vi "jeti_radio_ex64.vi"() -> ()   [LabVIEW 2018]
uses:
  C:/Windows/System32/jeti_radio_ex64.dll
panel:
  out "?":u16
  out "?":u16
  out "DLL Version":u16
  out "Device":string
  out "y":sgl
  out "x":sgl
  out "Radiometric Value":sgl
  out "Waveform Graph":cluster{dbl, dbl, "fDark":sgl[]}(graph)
  in  "Integration Time [ms]":sgl max=65000 step=1
  out "Device connected":bool
  in  "Measurement":bool
  out "dwDevice":u64
  in  "QuitButton":bool
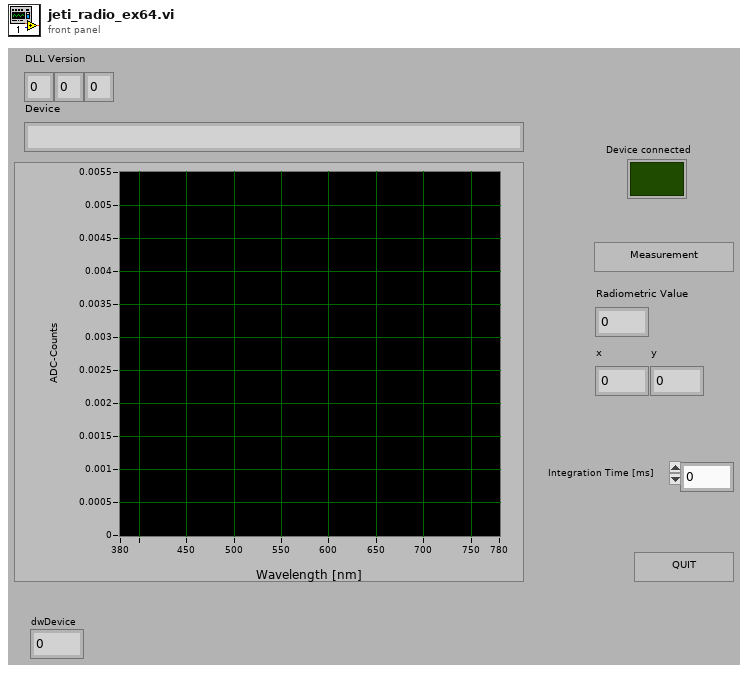
[diagram p1: front panel]
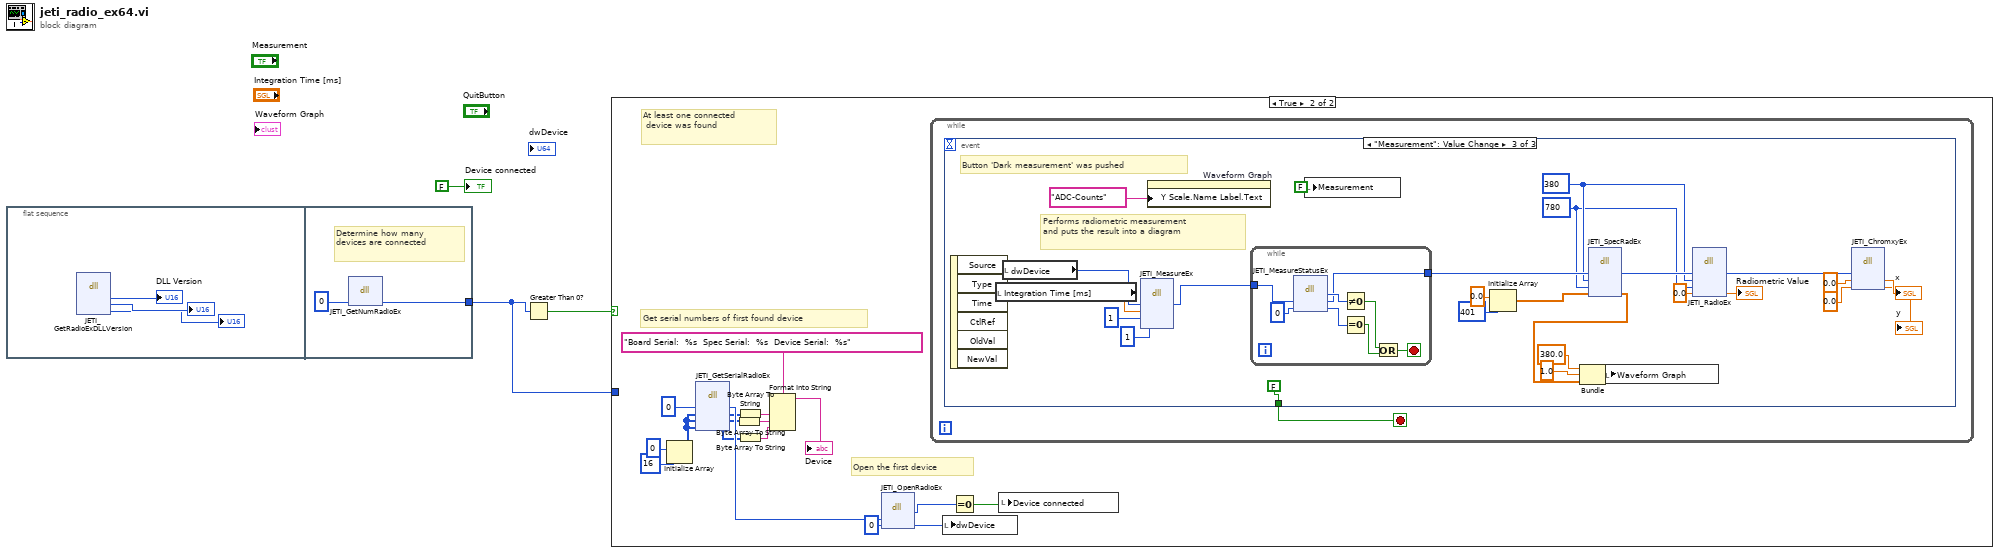
[diagram p0: block diagram]
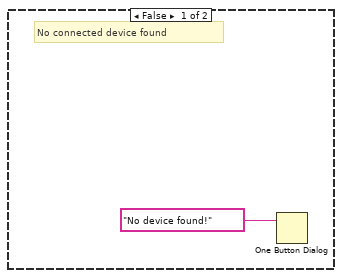
[diagram p2: hidden frame]
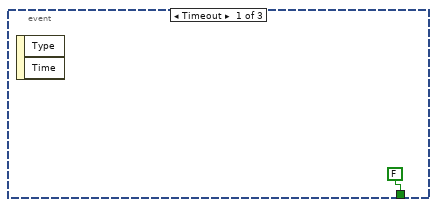
[diagram p3: hidden frame]
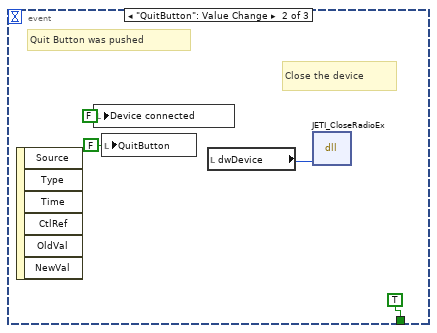
[diagram p4: hidden frame]
diagram:
  n1 = flat-sequence {
    tunnel: [w7] -> w1
    frame #0 {
      n2 = dll-call lib="C:/Windows/System32/jeti_radio_ex64.dll" fn="JETI_GetRadioExDLLVersion"() -> ("wMajorVersion"=→"DLL Version":u16, "wMinorVersion"=→"?":u16, "wBuildNumber"=→"?":u16)  [unwired: 7 in, 2 out]
    }
    frame #1 {
      # "Determine how many \ndevices are connected"
      n3 = dll-call lib="C:/Windows/System32/jeti_radio_ex64.dll" fn="JETI_GetNumRadioEx"("dwNumDevice"=u32 0) -> ("dwNumDevice"=w7:u32)  [unwired: 4 in, 2 out]
    }
  }
  n4 = Greater Than 0?(x=w1) -> (x > 0?=w3:bool)
  n5 = case shown="True" w3 {
    tunnel: w1 -> [_ _]
    frame False {
      # "No connected device found"
      n6 = One Button Dialog(message="No device found!") -> ()  [unwired: 1 in, 1 out]
    }
    frame True {
      # "Open the first device"
      # "Get serial numbers of first found device"
      # "At least one connected\n device was found"
      n7 = Initialize Array(i8 0 ("element"), 16 ("dimension size")) -> (w16:i8[])
      n8 = dll-call lib="C:/Windows/System32/jeti_radio_ex64.dll" fn="JETI_GetSerialRadioEx"("dwDeviceNum"=u32 0, "cBoardSerialNr"=w16, "cSpecSerialNr"=w16, "cDeviceSerialNr"=w16) -> ("dwDeviceNum"=w19:u32, "cBoardSerialNr"=w15:u8[], "cSpecSerialNr"=w13:u8[], "cDeviceSerialNr"=w11:u8[])  [unwired: 4 in, 2 out]
      n9 = Byte Array To String(unsigned byte array=w13) -> (string=w12:string)
      n10 = Byte Array To String(unsigned byte array=w15) -> (string=w14:string)
      n11 = Byte Array To String(unsigned byte array=w11) -> (string=w10:string)
      n12 = Format Into String(format string="Board Serial:  %s  Spec Serial:  %s  Device Serial:  %s", w14, w12, w10) -> (resulting string=→"Device":string)  [unwired: 2 in, 1 out]
      n13 = dll-call lib="C:/Windows/System32/jeti_radio_ex64.dll" fn="JETI_OpenRadioEx"("dwDeviceNum"=w19, "dwDevice"=u32 0) -> ("return type"=w22:u32, "dwDevice"=w21:u64)  [unwired: 4 in, 2 out]
      n14 = while {
        stop <- w27 stop-if-true
        n15 = event shown="[2] \"Measurement\": Value Change" {
          selector: _ -> [_ _ _]
          dyn-events: _ -> [_ _ _]
          timeout: _ -> [_ _ _]
          tunnel: [FALSE TRUE FALSE] -> w27
          event Timeout {
            n16 = event-data() -> ()  [unwired: 1 in, 2 out]
          }
          event "QuitButton": Value Change {
            # "Close the device"
            # "Quit Button was pushed"
            n17 = event-data() -> ()  [unwired: 1 in, 6 out]
            n18 = local write "Device connected"(FALSE ("Device connected")) -> ()
            n19 = local write "QuitButton"(FALSE ("QuitButton")) -> ()
            n20 = local read "dwDevice"() -> (w31:u64)
            n21 = dll-call lib="C:/Windows/System32/jeti_radio_ex64.dll" fn="JETI_CloseRadioEx"("dwDevice"=w31) -> ()  [unwired: 5 in, 2 out]
          }
          event "Measurement": Value Change {
            w37 = u32 780 ("dwEnd")
            w38 = u32 380 ("dwBeg")
            # "Button 'Dark measurement' was pushed"
            # "Performs radiometric measurement\nand puts the result into a diagram"
            n22 = event-data() -> ()  [unwired: 1 in, 6 out]
            n23 = local read "Integration Time [ms]"() -> (w56:sgl)
            n24 = local read "dwDevice"() -> (w57:u64)
            n25 = dll-call lib="C:/Windows/System32/jeti_radio_ex64.dll" fn="JETI_MeasureEx"("dwDevice"=w57, "fTint"=w56, "wAver"=u16 1, "dwStep"=u32 1) -> ("dwDevice"=w48:u64)  [unwired: 7 in, 2 out]
            n26 = property on="Waveform Graph" class="WFGraph (strict)"("Y Scale.Name Label.Text"="ADC-Counts") -> ()  [unwired: 2 in, 2 out]
            n27 = while {
              tunnel: w48 -> [w65]
              tunnel: [w59] -> w47
              stop <- w66 stop-if-true
              n28 = dll-call lib="C:/Windows/System32/jeti_radio_ex64.dll" fn="JETI_MeasureStatusEx"("dwDevice"=w65, "boStatus"=0) -> ("return type"=w63:u32, "dwDevice"=w59:u64, "boStatus"=w60:i32)  [unwired: 3 in, 2 out]
              n29 = Not Equal To 0?(x=w63) -> (x != 0?=w62:bool)
              n30 = Equal To 0?(x=w60) -> (x = 0?=w61:bool)
              n31 = Or(x=w62, y=w61) -> (x .or. y?=w66:bool)
            }
            n32 = local write "Measurement"(FALSE ("Dark")) -> ()
            n33 = Initialize Array(sgl 0.0 ("element"), 401 ("dimension size")) -> (w44:sgl[])
            n34 = dll-call lib="C:/Windows/System32/jeti_radio_ex64.dll" fn="JETI_SpecRadEx"("dwDevice"=w47, "dwBeg"=w38, "dwEnd"=w37, "fSprad"=w44) -> ("dwDevice"=w42:u64, "fSprad"=w43:sgl[])  [unwired: 6 in, 2 out]
            n35 = Bundle(380.0, 1.0, "fSprad"=w43) -> (w53:cluster{dbl, dbl, "fSprad":sgl[]})  [unwired: 1 in]
            n36 = local write "Waveform Graph"(w53) -> ()
            n37 = dll-call lib="C:/Windows/System32/jeti_radio_ex64.dll" fn="JETI_RadioEx"("dwDevice"=w42, "dwBeg"=w38, "dwEnd"=w37, "fRadio"=sgl 0.0) -> ("dwDevice"=w39:u64, "fRadio"=→"Radiometric Value":sgl)  [unwired: 6 in, 2 out]
            n38 = dll-call lib="C:/Windows/System32/jeti_radio_ex64.dll" fn="JETI_ChromxyEx"("dwDevice"=w39, "fChromX"=sgl 0.0, "fChromY"=sgl 0.0) -> ("fChromX"=→"x":sgl, "fChromY"=→"y":sgl)  [unwired: 5 in, 2 out]
          }
        }
      }
      n39 = local write "dwDevice"(w21) -> ()
      n40 = Equal To 0?(x=w22) -> (x = 0?=w23:bool)
      n41 = local write "Device connected"(w23) -> ()
    }
  }
  "Device connected" <- FALSE ("Device connected")
